vi "AlliGator Load Phasor Plots v3.vi"(8 "Error In":errorcluster, 10 "File paths":path[](array[path]) caption="selected paths", 11 "XYGraph in":refnum<vi>) -> (0 "Error Out":errorcluster, 1 "Last Raw Phasor Plot":cluster{"g":dbl[], "s":dbl[]}, 2 "Message":string, 3 "Raw Phasor Plot":T1[](array[typedef]) {"[Decay Metadata]"."# Folds" min=1; "[Decay Metadata]"."ROI Descriptor"."Contours"."Type" items=["No Selection", "Point", "Line", "Rectangle", "Oval", "Polygon", "Freehand Region", "Annulus", "Unused2", "Unused3", "Broken Line", "Freehand Line", "Rotated Rectangle"]})   [LabVIEW 2021, in "AlliGator Phasor Graph.lvlib"]
doc: "Loads Phasor Plot(s) and associated data and metadata from a phplot file.\n\nIf no file paths are provided, a dialog window is shown."
uses:
  AlliGator Phasor Graph.lvlib
  AlliGator Raw Phasor Plot Data v5.ctl
  Phasor/Phasor (g, s).ctl
  AlliGator Decay Metadata v3.ctl
  Decay Analysis/Decay Preprocessing/AlliGator Decay Background Subtraction Info.ctl
  Decay Analysis/Decay Preprocessing/AlliGator Baseline Subtraction Method.ctl
  Graphs/XY Graph/XY Graph Plot Shift Parameters.ctl
  Graphs/XY Graph/XY Graph Plot Shift Method.ctl
  Decay Analysis/Decay Preprocessing/AlliGator Decay Extrapolation Parameters.ctl
  Phasor/Phasor Standard Deviation Options.ctl
  Phasor/Calibration Phasor (m, phi).ctl
  Graphs/LabVIEW Plot Interpolation.ctl
  Graphs/Plot Point Style.ctl
  AlliGator Raw Phasor Plot Data v2.ctl
  AlliGator Decay Metadata.ctl
  AlliGator Raw Phasor Plot Data v1.ctl
  AlliGator Raw Phasor Plot Data v3.ctl
  AlliGator Raw Phasor Plot Data v4.ctl
  d75a8ec3-395c-45c9-858a-6d0515c4ea0f.vi
  4623fcf5-0913-4af6-b274-a61fc63dc5a4.vi
  068f6334-c7bc-4b58-b106-ea81d4237ab9.vi
  0c853f4a-822e-4e08-953f-69121264586e.vi
  9735f987-b6b5-414e-80a6-54cad8db5d94.vi
  <vilib>/Utility/error.llb/Error Cluster From Error Code.vi
  <vilib>/JDP Science/JSONtext/JSON text to Variant.vi
  Utilities/Logical Processors Used.vi
  Graphs/XY Graph/XY Graph Add Single Plot with Name.vi
  <vilib>/ErrorRing/Error Ring.xnode
  <vilib>/JDP Science/JSONtext/LVClass Serializer/JSONtext LVClass Serializer.lvclass
  Graphs/XY Graph/XY Graph Add-Ons.lvlib
  Phasor/Phasor.lvlib
  Files/Files.lvlib
  Graphs/Graphs.lvlib
  Decay Analysis/Decay Preprocessing/AlliGator Decay Preprocessing.lvlib
  Strings/Strings.lvlib
panel:
  # "see the License on the block diagram (Ctrl+E or Window:Show Block Diagram)"
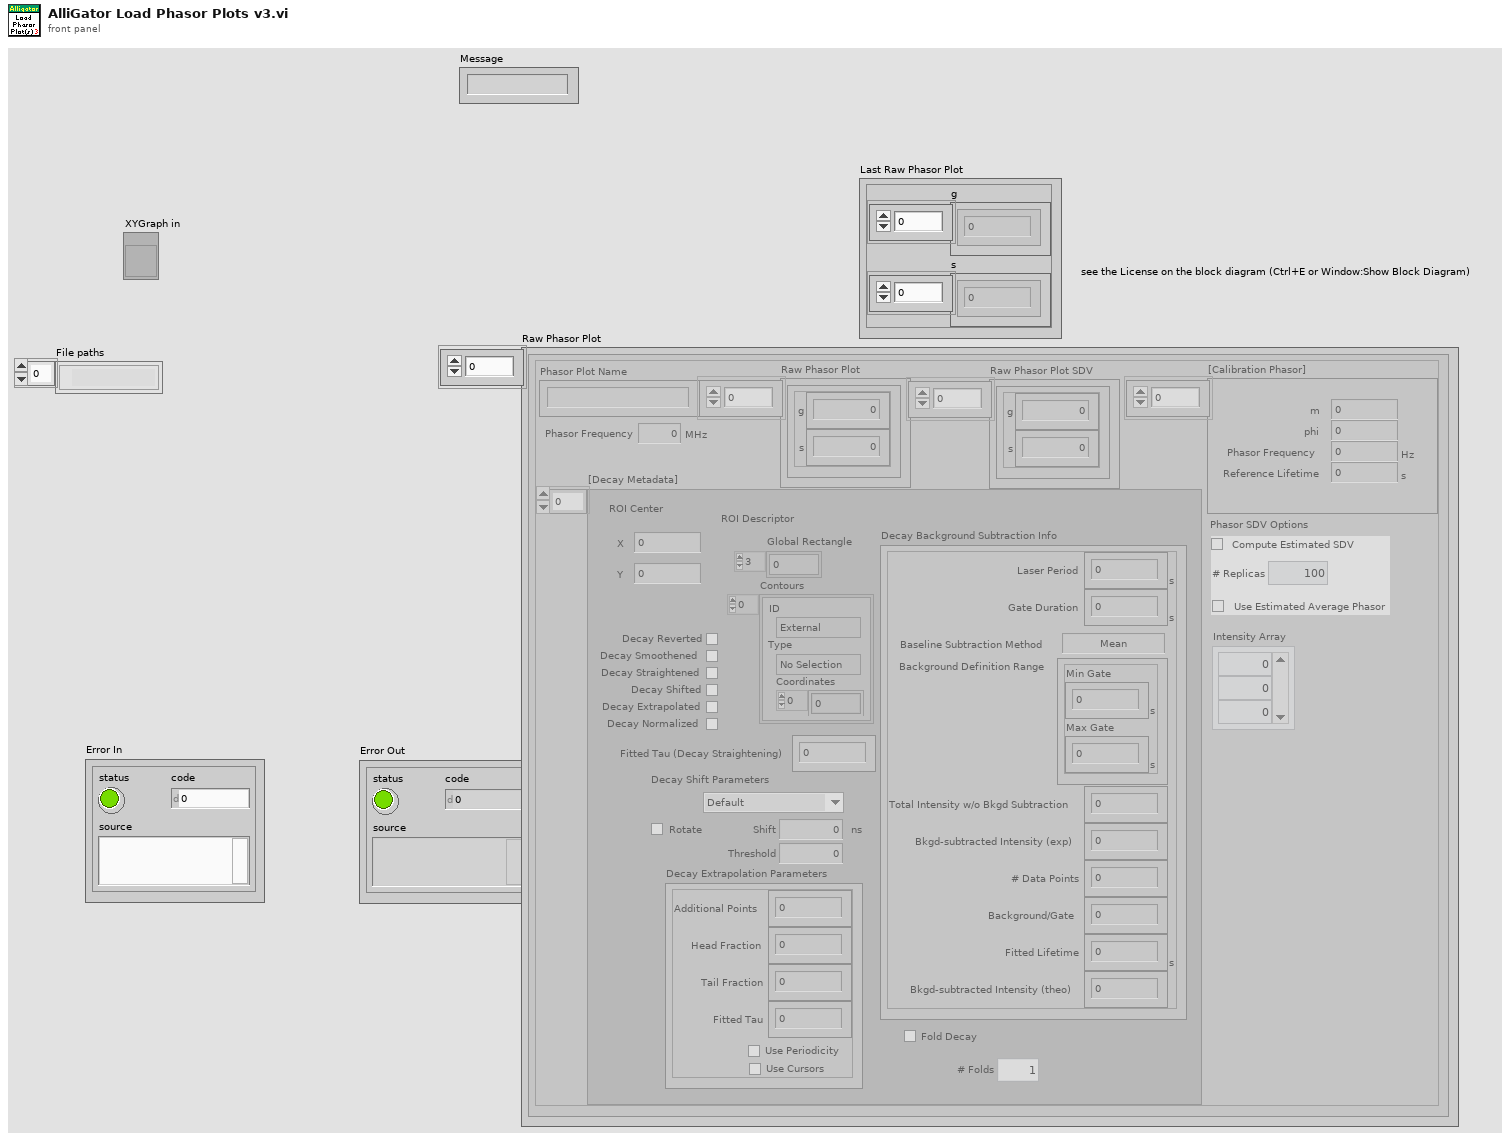
[diagram p1: front panel]
types:
  T1 = typedef "AlliGator Phasor Graph.lvlib/AlliGator Raw Phasor Plot Data v5.ctl" = cluster{"Phasor Plot Name":string, "Raw Phasor Plot":T2[], "Phasor Frequency":dbl[unit], "[Decay Metadata]":T3[], "Raw Phasor Plot SDV":T2[], "Phasor SDV Options":T10, "[Calibration Phasor]":T11[], "Intensity Array":dbl[]}
  T2 = typedef "Phasor.lvlib/Phasor (g, s).ctl" = cluster{"g":dbl, "s":dbl}
  T3 = typedef "AlliGator Phasor Graph.lvlib/AlliGator Decay Metadata v3.ctl" = cluster{"ROI Descriptor":T4, "ROI Center":cluster{"X":i32, "Y":i32}, "Decay Background Subtraction Info":T5, "Decay Reverted":bool, "Decay Smoothened":bool, "Decay Straightened":bool, "Fitted Tau (Decay Straightening)":dbl, "Decay Shift Parameters":T7, "Decay Shifted":bool, "Decay Extrapolated":bool, "Decay Extrapolation Parameters":T9, "Decay Normalized":bool, "Fold Decay":bool, "# Folds":u32}
  T4 = typedef "ROI Descriptor" = cluster{"Global Rectangle":i32[], "Contours":cluster{"ID":enum32{"External", "Internal"}, "Type":u32, "Coordinates":i32[]}[]}
  T5 = typedef "AlliGator Decay Preprocessing.lvlib/AlliGator Decay Background Subtraction Info.ctl" = cluster{"Laser Period":dbl[unit], "Gate Duration":dbl[unit], "Baseline Subtraction Method":T6, "Background Definition Range":cluster{"Min Gate":dbl[unit], "Max Gate":dbl[unit]}, "Total Intensity w/o Bkgd Subtraction":dbl, "Bkgd-subtracted Intensity (exp)":dbl, "# Data Points":i32, "Background/Gate":dbl, "Fitted Lifetime":dbl[unit], "Bkgd-subtracted Intensity (theo)":dbl}
  T6 = typedef "AlliGator Decay Preprocessing.lvlib/AlliGator Baseline Subtraction Method.ctl" = enum16{"Mean", "Min", "Square Gated Single-Exponential", "File", "Constant"}
  T7 = typedef "XY Graph Add-Ons.lvlib/XY Graph Plot Shift Parameters.ctl" = cluster{"Type":T8, "Shift":dbl[unit], "Threshold":dbl, "Rotate":bool}
  T8 = typedef "XY Graph Add-Ons.lvlib/XY Graph Plot Shift Method.ctl" = enum16{"Default", "CFD", "Threshold", "Cross-Correlation"}
  T9 = typedef "AlliGator Decay Preprocessing.lvlib/AlliGator Decay Extrapolation Parameters.ctl" = cluster{"Additional Points":u32, "Head Fraction":dbl, "Fitted Tau":dbl, "Use Periodicity":bool, "Use Cursors":bool, "Tail Fraction":dbl}
  T10 = typedef "Phasor.lvlib/Phasor Standard Deviation Options.ctl" = cluster{"Compute Estimated SDV":bool, "# Replicas":u32, "Use Estimated Average Phasor":bool}
  T11 = typedef "Phasor.lvlib/Calibration Phasor (m, phi).ctl" = cluster{"m":dbl, "phi":dbl, "Phasor Frequency":dbl[unit], "Reference Lifetime":dbl[unit]}
  T12 = typedef "Graphs.lvlib/Plot Point Style.ctl" = enum16{"not defined", "None", "Empty Circle", "Filled Circle", "Thick Circle", "Dotted Circle", "Empty Square", "Filled Square", "Thick Square", "Dotted Square", "Small Filled Square", "Dot", "Cross", "Tiny Cross", "Large X", "Small x", "Diamond", "Small Empty Square"}
  T13 = typedef "Graphs.lvlib/LabVIEW Plot Interpolation.ctl" = enum16{"Point (.)", "Stepwise Right (--.)", "Line + Point (\\. /)", "Stepwise Left (.--)", "Stepwise Centered (-.-)", "Stepwise Vertical (|.|)", "Line (-)", "Use Previous Plot's Style"}
  T14 = typedef "AlliGator Phasor Graph.lvlib/AlliGator Raw Phasor Plot Data v2.ctl" = cluster{"Plot Name":string, "Raw Phasor Plot":T2[], "Phasor Frequency":dbl[unit], "Phasor Metadata":T15[]}
  T15 = typedef "AlliGator Phasor Graph.lvlib/AlliGator Decay Metadata.ctl" = cluster{"Total Intensity":dbl, "# Gates":i32, "Background":dbl, "Amplitude":dbl, "Lifetime":dbl[unit], "Bkgd-subtracted Intensity (exp)":dbl, "Bkgd-subtracted Intensity (theo)":dbl}
  T16 = typedef "AlliGator Phasor Graph.lvlib/AlliGator Raw Phasor Plot Data v1.ctl" = cluster{"Plot Name":string, "Raw Phasor Plot":T2[], "Phasor Frequency":dbl[unit]}
  T17 = typedef "AlliGator Phasor Graph.lvlib/AlliGator Raw Phasor Plot Data v3.ctl" = cluster{"Plot Name":string, "Raw Phasor Plot":T2[], "Phasor Frequency":dbl[unit], "Phasor Metadata":T3[]}
  T18 = typedef "AlliGator Phasor Graph.lvlib/AlliGator Raw Phasor Plot Data v4.ctl" = cluster{"Phasor Plot Name":string, "Raw Phasor Plot":T2[], "Phasor Frequency":dbl[unit], "[Decay Metadata]":T3[], "Raw Phasor Plot SDV":T2[], "Phasor SDV Options":T10, "[Calibration Phasor]":T11[]}
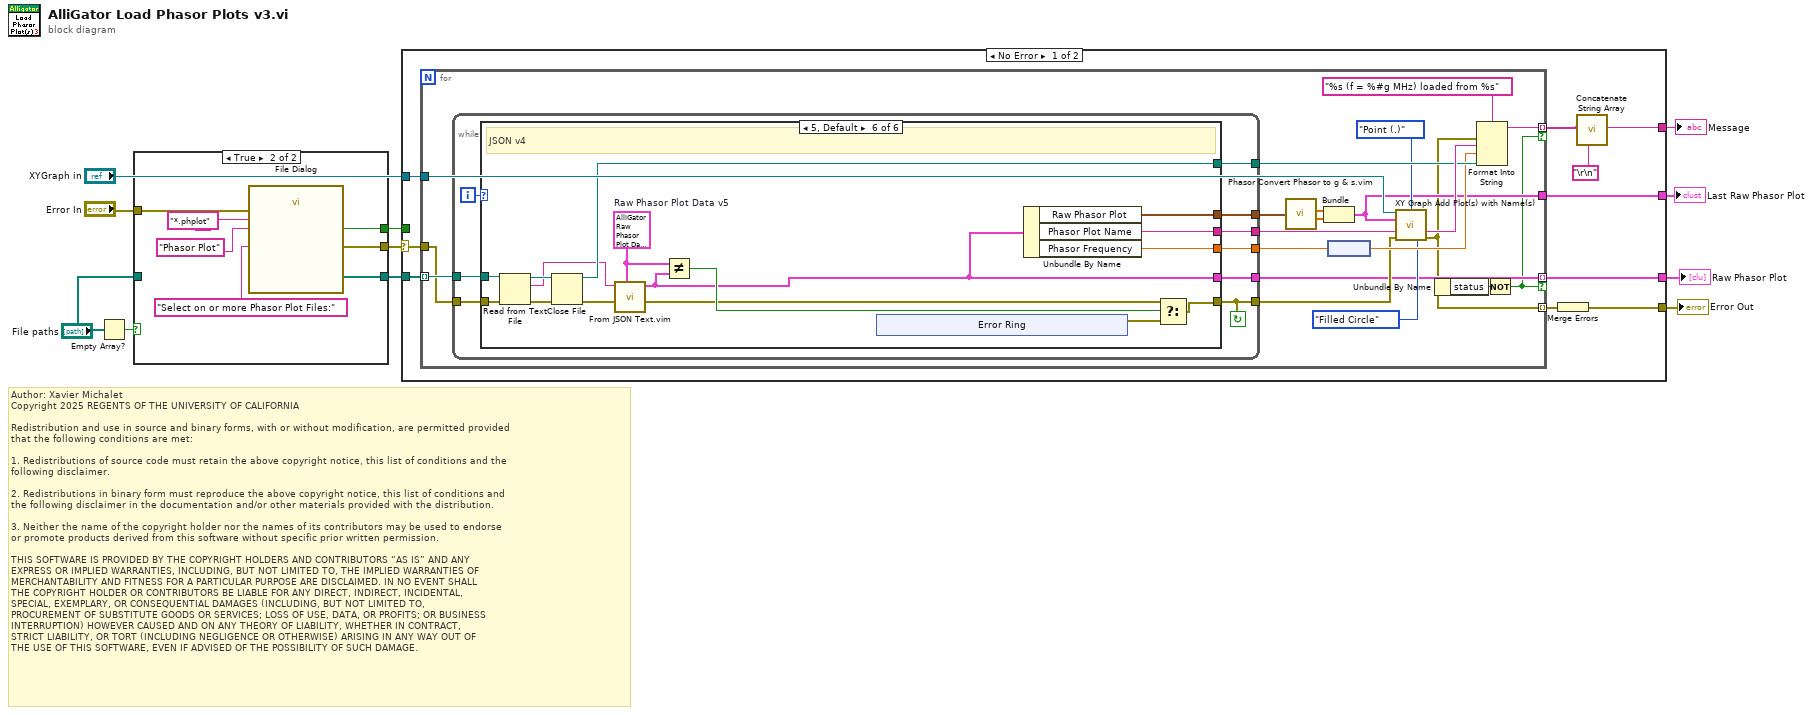
[diagram p0: block diagram]
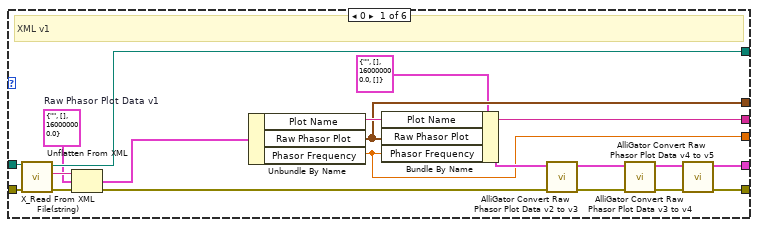
[diagram p3: hidden frame]
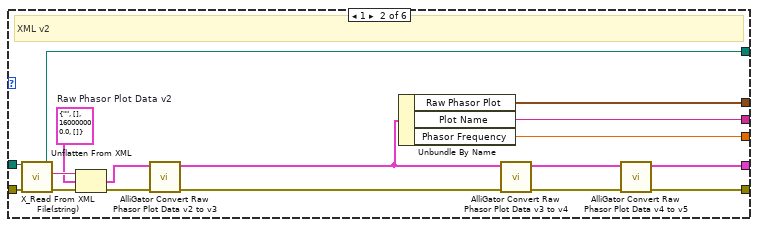
[diagram p4: hidden frame]
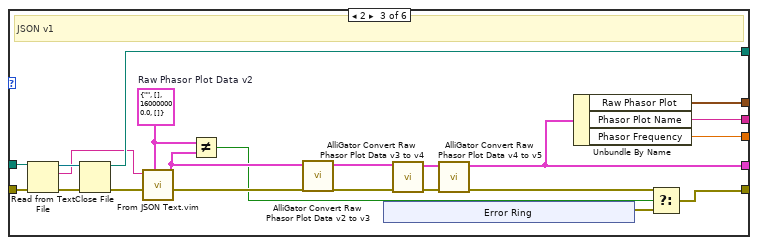
[diagram p5: hidden frame]
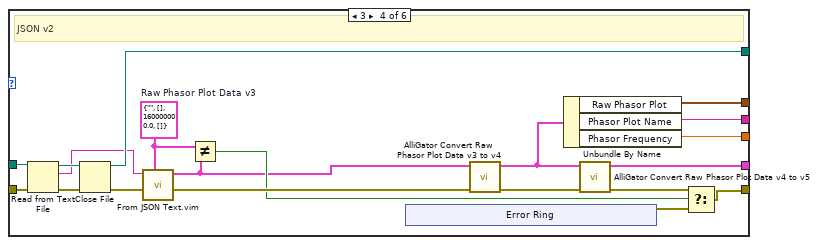
[diagram p6: hidden frame]
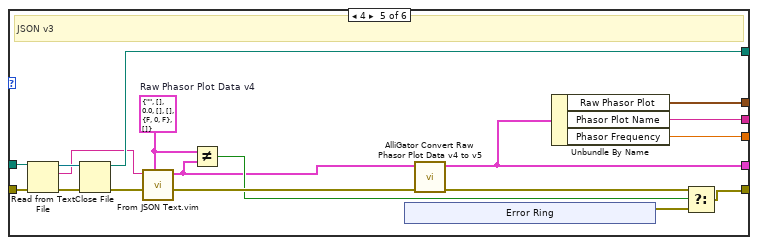
[diagram p7: hidden frame]
diagram:
  # "Author: Xavier Michalet\nCopyright 2025 REGENTS OF THE UNIVERSITY OF CALIFORNIA\n\nRedistribution and use in source and binary forms, with or without modification, are permitted provided\nthat the following conditions are met:\n\n1. Redistributions of source code must retain the above copyright notice, this list of conditions and the\nfollowing disclaimer.\n\n2. Redistributions in binary form must reproduce the above copyright notice, this list of conditions and\nthe following disclaimer in the documentation and/or other materials provided with the distribution.\n\n3. Neither the name of the copyright holder nor the names of its contributors may be used to endorse \nor promote products derived from this software without specific prior written permission.\n\nTHIS SOFTWARE IS PROVIDED BY THE COPYRIGHT HOLDERS AND CONTRIBUTORS “AS IS” AND ANY \nEXPRESS OR IMPLIED WARRANTIES, INCLUDING, BUT NOT LIMITED TO, THE IMPLIED WARRANTIES OF\nMERCHANTABILITY AND FITNESS FOR A PARTICULAR PURPOSE ARE DISCLAIMED. IN NO EVENT SHALL\nTHE COPYRIGHT HOLDER OR CONTRIBUTORS BE LIABLE FOR ANY DIRECT, INDIRECT, INCIDENTAL, \nSPECIAL, EXEMPLARY, OR CONSEQUENTIAL DAMAGES (INCLUDING, BUT NOT LIMITED TO, \nPROCUREMENT OF SUBSTITUTE GOODS OR SERVICES; LOSS OF USE, DATA, OR PROFITS; OR BUSINESS\nINTERRUPTION) HOWEVER CAUSED AND ON ANY THEORY OF LIABILITY, WHETHER IN CONTRACT, \nSTRICT LIABILITY, OR TORT (INCLUDING NEGLIGENCE OR OTHERWISE) ARISING IN ANY WAY OUT OF\nTHE USE OF THIS SOFTWARE, EVEN IF ADVISED OF THE POSSIBILITY OF SUCH DAMAGE."
  n1 = Empty Array?(array="File paths") -> (empty?=w3:bool)
  n2 = case shown="True" w3 {
    tunnel: [w13 w20] -> w9
    tunnel: [w12 w19] -> w8
    tunnel: [_ w18] -> w7
    tunnel: "Error In" -> [w12 w17]
    tunnel: "File paths" -> [w13 _]
    frame False {
    }
    frame True {
      n3 = call "File Dialog"("prompt"="Select on or more Phasor Plot Files:", "error in"=w17, "pattern (all files)"="*.phplot" ("pattern (*.phplot)"), "pattern label"="Phasor Plot") -> ("selected paths"=w20:path[], "cancelled"=w18:bool, "error out"=w19:errorcluster)  [unwired: 8 in, 1 out]
    }
  }
  n4 = case shown="No Error" w8 {
    selector: w8 -> [w26 _]
    tunnel: "XYGraph in" -> [w30 _]
    tunnel: [w28 _] -> w10
    tunnel: w9 -> [w27 _]
    tunnel: [w25 _] -> w5
    tunnel: [w24 _] -> w4
    tunnel: w7 -> [_ _]
    tunnel: [w21 _] -> w1
    frame No Error {
      n5 = for {
        tunnel: w27 -> [w50] mode=indexing
        tunnel: w30 -> [w51]
        tunnel: [w33] -> w29 mode=indexing
        tunnel: w26 -> [w49]
        tunnel: [w34] -> w25 mode=indexing if=w31
        tunnel: [w36] -> w24
        tunnel: [w32] -> w23 mode=indexing if=w31
        n6 = while {
          tunnel: [w58] -> w48
          tunnel: [w57] -> w47
          tunnel: [w55] -> w41
          tunnel: [w54] -> w34
          tunnel: w50 -> [w60]
          tunnel: [w56] -> w42
          tunnel: w49 -> [w59]
          tunnel: [w53] -> w35
          i -> [w52]
          stop <- w53 continue-if-true
          n7 = case shown="5, Default" w52 {
            tunnel: w60 -> [w79 w96 w113 w140 w162 w182]
            tunnel: w59 -> [w78 w95 w114 w141 w163 w183]
            tunnel: [w77 w94 w117 w126 w151 w172] -> w58
            tunnel: [w76 w93 w116 w127 w152 w173] -> w57
            tunnel: [w75 w92 w110 w137 w159 w179] -> w56
            tunnel: [w64 w91 w115 w125 w150 w171] -> w55
            tunnel: [w61 w81 w97 w122 w146 w169] -> w54
            tunnel: [w63 w82 w100 w133 w155 w176] -> w53
            frame 0 {
              w71 = T16 {"Plot Name"="", "Raw Phasor Plot"=[], "Phasor Frequency"=160000000.0}  # Raw Phasor Plot Data v1
              # "XML v1"
              n8 = call "X_Read From XML File(string).vi"("error in (no error)"=w78, "XML File Path"=w79) -> ("error out"=w73:errorcluster, "XML Elements"=w74:string, "XML File Path(duplicate)"=w75:path)  [unwired: 7 in]
              n9 = Unflatten From XML(xml string=w74, type=w71, error in (no error)=w73) -> (value=w70:T16, error out=w67:errorcluster)
              n10 = Unbundle By Name(w70) -> ("Plot Name"=w77:string, "Raw Phasor Plot"=w76:T2[], "Phasor Frequency"=w64:dbl[unit])
              n11 = Bundle By Name(cluster=T14 {"Plot Name"="", "Raw Phasor Plot"=[], "Phasor Frequency"=160000000.0, "Phasor Metadata"=[]} ("Raw Phasor Plot Data"), "Plot Name"=w77, "Raw Phasor Plot"=w76, "Phasor Frequency"=w64) -> (w66:T14)
              n12 = call "AlliGator Convert Raw Phasor Plot Data v2 to v3.vi"("Error In"=w67, "Raw Phasor Plot Data v2"=w66) -> ("Error Out"=w68:errorcluster, "Raw Phasor Plot Data v3"=w69:T17)  [unwired: 8 in]
              n13 = call "AlliGator Convert Raw Phasor Plot Data v3 to v4.vi"("error in (no error)"=w68, "Raw Phasor Plot Data v3"=w69) -> ("error out"=w65:errorcluster, "Raw Phasor Plot Data v4"=w62:T18)  [unwired: 8 in]
              n14 = call "AlliGator Convert Raw Phasor Plot Data v4 to v5.vi"("error in (no error)"=w65, "Raw Phasor Plot Data v4"=w62) -> ("error out"=w63:errorcluster, "Raw Phasor Plot Data v5"=w61:T1)  [unwired: 8 in]
            }
            frame 1 {
              w88 = T14 {"Plot Name"="", "Raw Phasor Plot"=[], "Phasor Frequency"=160000000.0, "Phasor Metadata"=[]}  # Raw Phasor Plot Data v2
              # "XML v2"
              n15 = call "X_Read From XML File(string).vi"("error in (no error)"=w95, "XML File Path"=w96) -> ("error out"=w89:errorcluster, "XML Elements"=w90:string, "XML File Path(duplicate)"=w92:path)  [unwired: 7 in]
              n16 = Unflatten From XML(xml string=w90, type=w88, error in (no error)=w89) -> (value=w87:T14, error out=w86:errorcluster)
              n17 = call "AlliGator Convert Raw Phasor Plot Data v2 to v3.vi"("Error In"=w86, "Raw Phasor Plot Data v2"=w87) -> ("Error Out"=w85:errorcluster, "Raw Phasor Plot Data v3"=w83:T17)  [unwired: 8 in]
              n18 = Unbundle By Name(w83) -> ("Raw Phasor Plot"=w93:T2[], "Plot Name"=w94:string, "Phasor Frequency"=w91:dbl[unit])
              n19 = call "AlliGator Convert Raw Phasor Plot Data v3 to v4.vi"("error in (no error)"=w85, "Raw Phasor Plot Data v3"=w83) -> ("error out"=w84:errorcluster, "Raw Phasor Plot Data v4"=w80:T18)  [unwired: 8 in]
              n20 = call "AlliGator Convert Raw Phasor Plot Data v4 to v5.vi"("error in (no error)"=w84, "Raw Phasor Plot Data v4"=w80) -> ("error out"=w82:errorcluster, "Raw Phasor Plot Data v5"=w81:T1)  [unwired: 8 in]
            }
            frame 2 {
              w105 = T14 {"Plot Name"="", "Raw Phasor Plot"=[], "Phasor Frequency"=160000000.0, "Phasor Metadata"=[]}  # Raw Phasor Plot Data v2
              # "JSON v1"
              n21 = Read from Text File(file (use dialog)=w113, error in=w114) -> (refnum out=w112:refnum<file>, text=w109:string, error out=w111:errorcluster)  [unwired: 2 in, 1 out]
              n22 = Close File(refnum=w112, error in=w111) -> (path=w110:path, error out=w108:errorcluster)
              n23 = call "From JSON Text.vim"("Data Type and Default Value"=w105, "error in (no error)"=w108, "JSON"=w109) -> ("error out"=w107:errorcluster, "Data out"=w104:T14)  [unwired: 7 in]
              n24 = Not Equal?(x=w105, y=w104) -> (x != y?=w101:bool)
              n25 = call "AlliGator Convert Raw Phasor Plot Data v2 to v3.vi"("Raw Phasor Plot Data v2"=w104) -> ("Raw Phasor Plot Data v3"=w106:T17)  [unwired: 9 in, 1 out]
              n26 = xnode "Error Ring"() -> ("error out"=w102:errorcluster)
              n27 = call "AlliGator Convert Raw Phasor Plot Data v3 to v4.vi"("error in (no error)"=w107, "Raw Phasor Plot Data v3"=w106) -> ("error out"=w103:errorcluster, "Raw Phasor Plot Data v4"=w98:T18)  [unwired: 8 in]
              n28 = call "AlliGator Convert Raw Phasor Plot Data v4 to v5.vi"("error in (no error)"=w103, "Raw Phasor Plot Data v4"=w98) -> ("error out"=w99:errorcluster, "Raw Phasor Plot Data v5"=w97:T1)  [unwired: 8 in]
              n29 = Unbundle By Name(w97) -> ("Raw Phasor Plot"=w116:T2[], "Phasor Plot Name"=w117:string, "Phasor Frequency"=w115:dbl[unit])
              n30 = Select(t=w99, s=w101, f=w102) -> (s? t:f=w100:errorcluster)
            }
            frame 3 {
              w130 = T17 {"Plot Name"="", "Raw Phasor Plot"=[], "Phasor Frequency"=160000000.0, "Phasor Metadata"=[]}  # Raw Phasor Plot Data v3
              # "JSON v2"
              n31 = Read from Text File(file (use dialog)=w140, error in=w141) -> (refnum out=w139:refnum<file>, text=w136:string, error out=w138:errorcluster)  [unwired: 2 in, 1 out]
              n32 = Close File(refnum=w139, error in=w138) -> (path=w137:path, error out=w135:errorcluster)
              n33 = call "From JSON Text.vim"("Data Type and Default Value"=w130, "error in (no error)"=w135, "JSON"=w136) -> ("error out"=w134:errorcluster, "Data out"=w128:T17)  [unwired: 7 in]
              n34 = Not Equal?(x=w130, y=w128) -> (x != y?=w129:bool)
              n35 = xnode "Error Ring"() -> ("error out"=w132:errorcluster)
              n36 = call "AlliGator Convert Raw Phasor Plot Data v3 to v4.vi"("error in (no error)"=w134, "Raw Phasor Plot Data v3"=w128) -> ("error out"=w131:errorcluster, "Raw Phasor Plot Data v4"=w123:T18)  [unwired: 8 in]
              n37 = Unbundle By Name(w123) -> ("Raw Phasor Plot"=w127:T2[], "Phasor Plot Name"=w126:string, "Phasor Frequency"=w125:dbl[unit])
              n38 = call "AlliGator Convert Raw Phasor Plot Data v4 to v5.vi"("error in (no error)"=w131, "Raw Phasor Plot Data v4"=w123) -> ("error out"=w124:errorcluster, "Raw Phasor Plot Data v5"=w122:T1)  [unwired: 8 in]
              n39 = Select(t=w124, s=w129, f=w132) -> (s? t:f=w133:errorcluster)
            }
            frame 4 {
              w149 = T18 {"Phasor Plot Name"="", "Raw Phasor Plot"=[], "Phasor Frequency"=0.0, "[Decay Metadata]"=[], "Raw Phasor Plot SDV"=[], "Phasor SDV Options"={"Compute Estimated SDV"=FALSE, "# Replicas"=0, "Use Estimated Average Phasor"=FALSE}, "[Calibration Phasor]"=[]}  # Raw Phasor Plot Data v4
              # "JSON v3"
              n40 = Read from Text File(file (use dialog)=w162, error in=w163) -> (refnum out=w161:refnum<file>, text=w158:string, error out=w160:errorcluster)  [unwired: 2 in, 1 out]
              n41 = Close File(refnum=w161, error in=w160) -> (path=w159:path, error out=w157:errorcluster)
              n42 = call "From JSON Text.vim"("Data Type and Default Value"=w149, "error in (no error)"=w157, "JSON"=w158) -> ("error out"=w156:errorcluster, "Data out"=w147:T18)  [unwired: 7 in]
              n43 = Not Equal?(x=w149, y=w147) -> (x != y?=w153:bool)
              n44 = xnode "Error Ring"() -> ("error out"=w154:errorcluster)
              n45 = call "AlliGator Convert Raw Phasor Plot Data v4 to v5.vi"("error in (no error)"=w156, "Raw Phasor Plot Data v4"=w147) -> ("error out"=w148:errorcluster, "Raw Phasor Plot Data v5"=w146:T1)  [unwired: 8 in]
              n46 = Unbundle By Name(w146) -> ("Raw Phasor Plot"=w152:T2[], "Phasor Plot Name"=w151:string, "Phasor Frequency"=w150:dbl[unit])
              n47 = Select(t=w148, s=w153, f=w154) -> (s? t:f=w155:errorcluster)
            }
            frame 5, Default {
              w170 = T1 {"Phasor Plot Name"="", "Raw Phasor Plot"=[], "Phasor Frequency"=160000000.0, "[Decay Metadata]"=[], "Raw Phasor Plot SDV"=[], "Phasor SDV Options"={"Compute Estimated SDV"=FALSE, "# Replicas"=100, "Use Estimated Average Phasor"=FALSE}, "[Calibration Phasor]"=[], "Intensity Array"=[]}  # Raw Phasor Plot Data v5
              # "JSON v4"
              n48 = Read from Text File(file (use dialog)=w182, error in=w183) -> (refnum out=w181:refnum<file>, text=w178:string, error out=w180:errorcluster)  [unwired: 2 in, 1 out]
              n49 = Close File(refnum=w181, error in=w180) -> (path=w179:path, error out=w177:errorcluster)
              n50 = call "From JSON Text.vim"("Data Type and Default Value"=w170, "error in (no error)"=w177, "JSON"=w178) -> ("error out"=w168:errorcluster, "Data out"=w169:T1)  [unwired: 7 in]
              n51 = Not Equal?(x=w170, y=w169) -> (x != y?=w174:bool)
              n52 = xnode "Error Ring"() -> ("error out"=w175:errorcluster)
              n53 = Unbundle By Name(w169) -> ("Raw Phasor Plot"=w173:T2[], "Phasor Plot Name"=w172:string, "Phasor Frequency"=w171:dbl[unit])
              n54 = Select(t=w168, s=w174, f=w175) -> (s? t:f=w176:errorcluster)
            }
          }
        }
        n55 = call "Phasor Convert Phasor to g & s.vim"("Phasor Array"=w47) -> ("g"=w46:dbl[], "s"=w45:dbl[])  [unwired: 8 in]
        n56 = Bundle("g"=w46, "s"=w45) -> (w36:cluster{"g":dbl[], "s":dbl[]})  [unwired: 1 in]
        n57 = node(w41) -> (w40:dbl)
        n58 = call-poly "XY Graph Add Plot(s) with Name(s).vi"("XYGraph Ref in"=w51, "Plot Interpolation (Previous Plot's Style)"=LabVIEW_Plot_Interpolation."Point (.)", "Plot"=w36, "Plot Name (\"Plot\")"=w48, "error in (no error)"=w35, "Point Style (Dot)"=Plot_Point_Style."Filled Circle") -> ("Plot Name"=w43:string, "error out"=w33:errorcluster)  [unwired: 6 in, 2 out]
        n59 = Unbundle By Name(w33) -> ("status"=w39:bool)
        n60 = Format Into String(format string="%s (f = %#g MHz) loaded from %s", error in=w33, w43, w40, w42) -> (resulting string=w32:string)  [unwired: 1 in, 1 out]
        n61 = Not(x=w39) -> (.not. x?=w31:bool)
      }
      n62 = Merge Errors(w29) -> (w28:errorcluster)
      n63 = call "Concatenate String Array.vi"("Separator (TAB)"="\r\n", "String Array"=w23) -> ("Formatted String"=w21:string)  [unwired: 9 in]
    }
    frame Error {
    }
  }
  "Error Out" <- w10
  "Raw Phasor Plot" <- w5
  "Last Raw Phasor Plot" <- w4
  "Message" <- w1
